vi "Example_guider.vi"() -> ()   [LabVIEW 2018]
panel:
  out "C":dbl
  in  "B":dbl
  in  "A":dbl
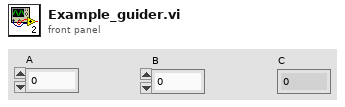
[diagram p1: front panel]
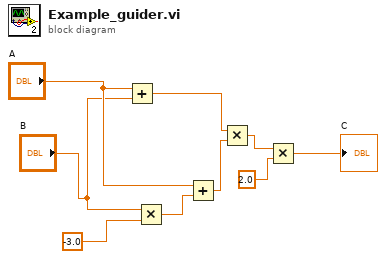
[diagram p0: block diagram]
diagram:
  n1 = Add(x="A", y="B") -> (x+y=w5:dbl)
  n2 = Multiply(x="B", y=-3.0 ("x")) -> (x*y=w7:dbl)
  n3 = Add(x="A", y=w7) -> (x+y=w4:dbl)
  n4 = Multiply(x=w5, y=w4) -> (x*y=w3:dbl)
  n5 = Multiply(x=w3, y=2.0 ("x")) -> (x*y=→"C":dbl)
